vi "写入名称.vi"(8 "error in (no error)":errorcluster caption="错误输入（无错误）", 10 "名称":string, 11 "鸭子输入":refnum<class "鸭子.lvclass">) -> (0 "error out":errorcluster caption="错误输出", 3 "鸭子输出":refnum<class "鸭子.lvclass">)   [LabVIEW 2022 SP3, in "鸭子库.lvlib" / "鸭子.lvclass"]
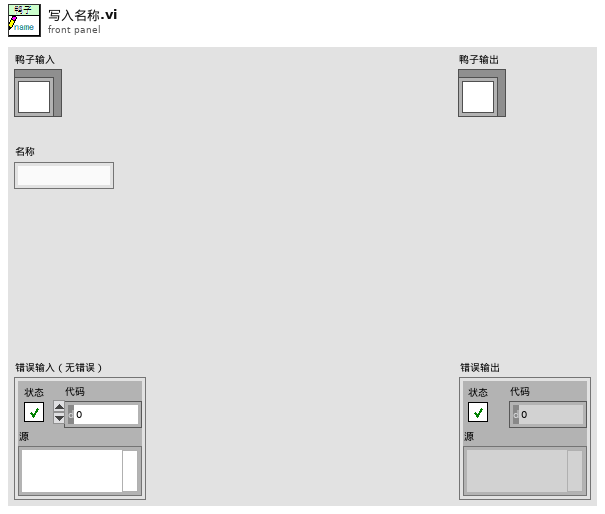
[diagram p1: front panel]
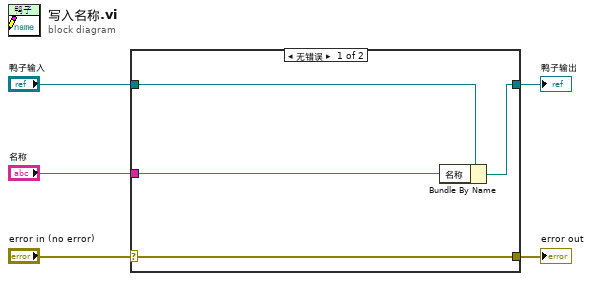
[diagram p0: block diagram]
diagram:
  n1 = case shown="无错误" "error in (no error)" {
    selector: "error in (no error)" -> [w9 w10]
    tunnel: [w9 w10] -> w4
    tunnel: [w7 w11] -> w2
    tunnel: "鸭子输入" -> [w8 w11]
    tunnel: "名称" -> [w6 _]
    frame No Error {
      n2 = Bundle By Name(cluster=w8, "名称"=w6) -> (w7:refnum<class "鸭子.lvclass">)
    }
    frame Error {
    }
  }
  "error out" <- w4
  "鸭子输出" <- w2
